vi "Build TS Activation Execution Plan.vi"(8 "error in":errorcluster, 11 "TSInstall":T2) -> (0 "error out":errorcluster, 3 "Execution Plan":T1={"Exe Path"=path "", "Args"=[], "Timeout"=-1})   [LabVIEW 2025]
doc: "This VI builds an execution plan to launch the TestStand Version Selector with specific arguments for activation or installation."
uses:
  Type Definitions/TSInstall--cluster.ctl
  Type Definitions/Architecture--enum.ctl
  Type Definitions/Execution Plan--cluster.ctl
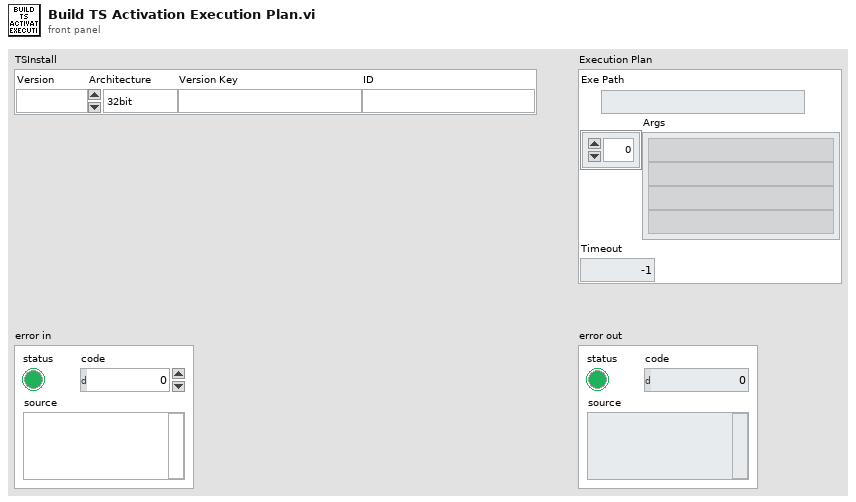
[diagram p1: front panel]
types:
  T1 = typedef "Execution Plan--cluster.ctl" = cluster{"Exe Path":path, "Args":string[], "Timeout":i32}
  T2 = typedef "TSInstall--cluster.ctl" = cluster{"Version":string, "Architecture":T3, "Version Key":string, "ID":string}
  T3 = typedef "Architecture--enum.ctl" = enum16{"32bit", "64bit"}
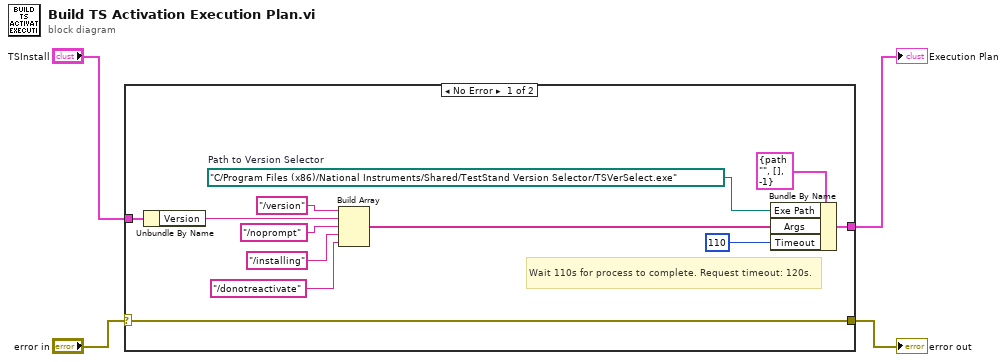
[diagram p0: block diagram]
diagram:
  n1 = case shown="No Error" "error in" {
    selector: "error in" -> [w13 w17]
    tunnel: "TSInstall" -> [w16 _]
    tunnel: [w14 _] -> w3
    tunnel: [w13 w17] -> w1
    frame No Error {
      w11 = path "C:/Program Files (x86)/National Instruments/Shared/TestStand Version Selector/TSVerSelect.exe"  # Path to Version Selector
      # "Wait 110s for process to complete. Request timeout: 120s."
      n2 = Unbundle By Name(w16) -> ("Version"=w9:string)
      n3 = Build Array("/version", w9, "/noprompt" ("element"), "/installing" ("element"), "/donotreactivate" ("element")) -> (w5:string[])
      n4 = Bundle By Name(cluster=T1 {"Exe Path"=path "", "Args"=[], "Timeout"=-1} ("Execution Plan"), "Exe Path"=w11, "Args"=w5, "Timeout"=110) -> (w14:T1)
    }
    frame Error {
      # "Pass error without further action"
    }
  }
  "Execution Plan" <- w3
  "error out" <- w1
